vi "Write Database.vi"(8 "error in (no error)":errorcluster, 10 "Database":variant, 11 "Message in":refnum<class "String Database.lvclass">=refnum) -> (0 "error out":errorcluster, 3 "Message out":refnum<class "String Database.lvclass">)   [LabVIEW 2018, in "String Database.lvlib" / "String Database.lvclass"]
uses:
  String Database.lvclass
  String Database.lvclass/String Database.ctl
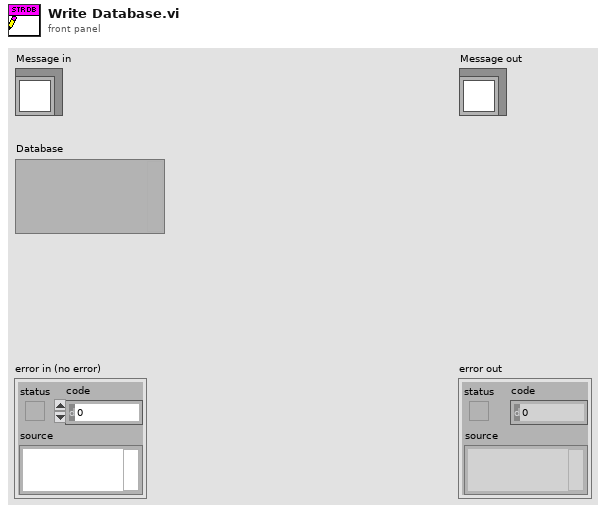
[diagram p1: front panel]
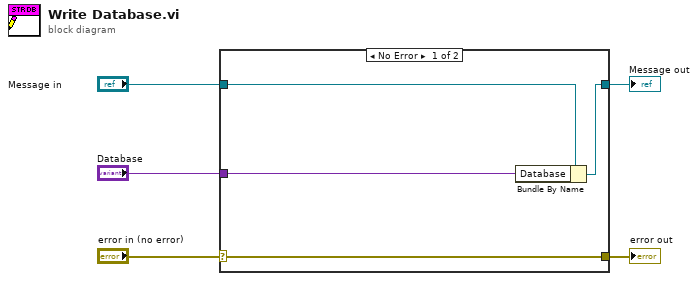
[diagram p0: block diagram]
diagram:
  n1 = case shown="No Error" "error in (no error)" {
    selector: "error in (no error)" -> [w9 w10]
    tunnel: [w9 w10] -> w4
    tunnel: [w7 w11] -> w2
    tunnel: "Message in" -> [w8 w11]
    tunnel: "Database" -> [w6 _]
    frame No Error {
      n2 = Bundle By Name(cluster=w8, "Database"=w6) -> (w7:refnum<class "String Database.lvclass">)
    }
    frame Error {
    }
  }
  "error out" <- w4
  "Message out" <- w2
